vi "Get Device Channels.vi"(8 "error in":errorcluster, 11 "Device Reference in":T1 format="%.0x") -> (0 "error out":errorcluster, 2 "Device Channels":T2 {"Status"."BD Refs"."Data Reference" format="%.0x"; "Command"."BD Refs"."Data Reference" format="%.0x"}, 3 "Device Reference out":T1 format="%.0x")   [LabVIEW 2020, in "SEECD Engine.lvlib"]
uses:
  SEECD Engine.lvlib
  <vilib>/NI VeriStand/Custom Device API/Custom Device Item Ref.ctl
  Type Defs/Device Channels.ctl
  Type Defs/Output Data.ctl
  <vilib>/NI VeriStand/Custom Device API/Block Data Reference.ctl
  <vilib>/NI VeriStand/Custom Device API/Data Reference.ctl
  Type Defs/Input Data.ctl
  Type Defs/Data Ref FGV Command.ctl
  <vilib>/NI VeriStand/Custom Device API/Custom Device Channel Type.ctl
  <vilib>/NI VeriStand/Custom Device API/Data Access Type.ctl
  <vilib>/NI VeriStand/Custom Device Tools/Custom Device Utility Library/NI VeriStand - Search for Item by Name.vi
  <vilib>/NI VeriStand/Custom Device Tools/Custom Device Utility Library/Custom Device Utility Library.lvlib
  <vilib>/NI VeriStand/Custom Device API/Custom Device API.lvlib
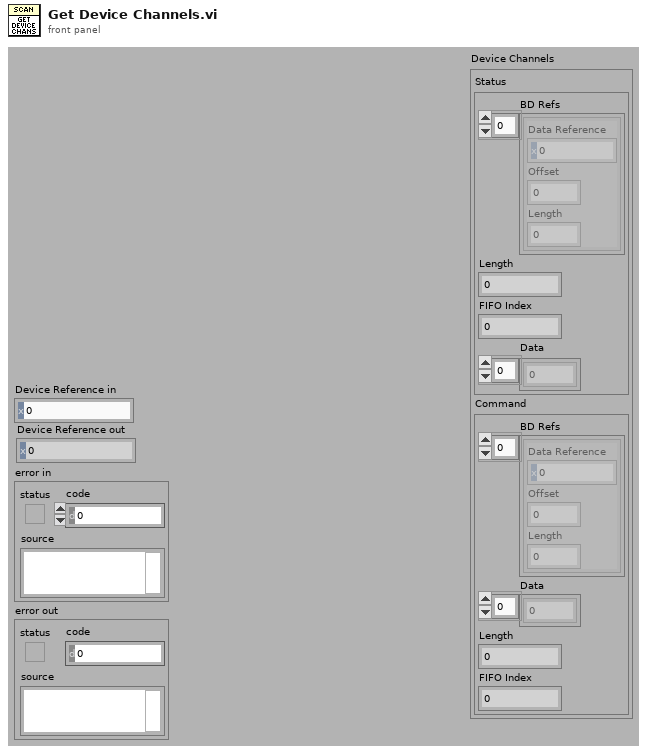
[diagram p1: front panel]
types:
  T1 = typedef "Custom Device API.lvlib/Custom Device Item Ref.ctl" = u64
  T2 = typedef "SEECD Engine.lvlib/Device Channels.ctl" = cluster{"Status":T3, "Command":T6}
  T3 = typedef "SEECD Engine.lvlib/Output Data.ctl" = cluster{"BD Refs":T4[], "Length":i32, "FIFO Index":i32, "Data":dbl[]}
  T4 = typedef "Custom Device API.lvlib/Block Data Reference.ctl" = cluster{"Data Reference":T5, "Offset":u64, "Length":u64}
  T5 = typedef "Custom Device API.lvlib/Data Reference.ctl" = i32
  T6 = typedef "SEECD Engine.lvlib/Input Data.ctl" = cluster{"BD Refs":T4[], "Data":dbl[], "Length":i32, "FIFO Index":i32}
  T7 = typedef "SEECD Engine.lvlib/Data Ref FGV Command.ctl" = enum16{"Intialize", "Get", "Update"}
  T8 = typedef "Custom Device API.lvlib/Data Access Type.ctl" = enum16{"Read", "Write"}
  T9 = typedef "Custom Device API.lvlib/Custom Device Channel Type.ctl" = enum16{"Input", "Output"}
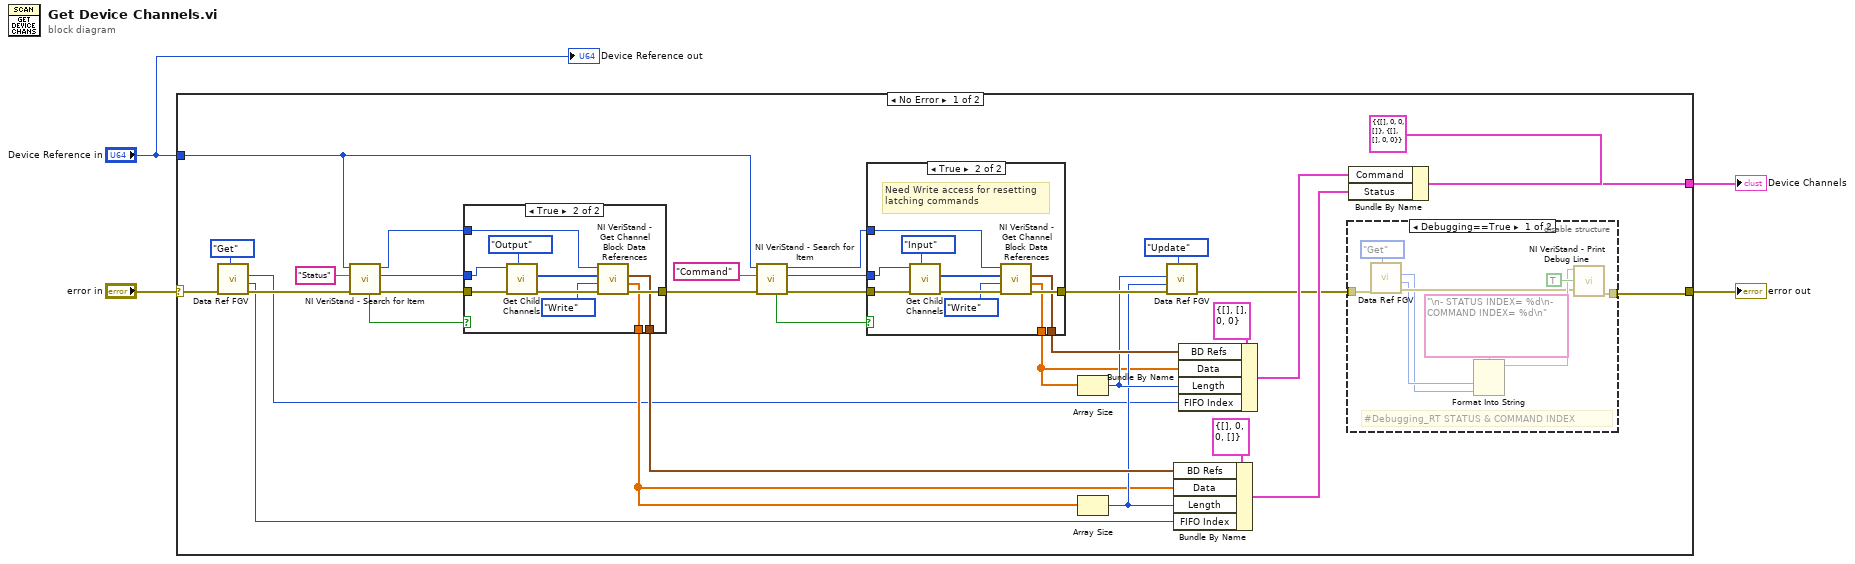
[diagram p0: block diagram]
diagram:
  n1 = case shown="No Error" "error in" {
    selector: "error in" -> [w28 w70]
    tunnel: [w5 w70] -> w3
    tunnel: "Device Reference in" -> [w31 _]
    tunnel: [w29 _] -> w1
    frame No Error {
      n2 = call "Data Ref FGV.vi"("Command"=Data_Ref_FGV_Command."Get", "error in (no error)"=w28) -> ("error out"=w27:errorcluster, "Output FIFO Index / Length"=w8:i32, "Input FIFO Index / Length"=w7:i32)  [unwired: 6 in, 1 out]
      n3 = call-poly <vilib>:"NI VeriStand - Search for Item.vi"("error in"=w27, "Item Name"="Status" ("Section Name"), "Section Ref in"=w31) -> ("error out"=w34:errorcluster, "Item Ref"=w35:T1, "Section Ref out"=w25:T1, "Found"=w36:bool)  [unwired: 5 in]
      n4 = case shown="True" w36 {
        tunnel: w35 -> [_ w68]
        tunnel: w34 -> [w59 w67]
        tunnel: [w59 w65] -> w30
        tunnel: w25 -> [_ w63]
        tunnel: [_ w61] -> w10
        tunnel: [_ w60] -> w18
        frame False {
        }
        frame True {
          n5 = call "Get Child Channels.vi"("Channel Type"=Custom_Device_Channel_Type."Output", "error in"=w67, "Section Ref in"=w68) -> ("error out"=w66:errorcluster, "Channel Refs"=w64:T1[])  [unwired: 5 in, 2 out]
          n6 = call <vilib>:"NI VeriStand - Get Channel Block Data References.vi"("error in (no error)"=w66, "Access"=Data_Access_Type."Write", "Channel Refs"=w64, "Device Ref in"=w63) -> ("error out"=w65:errorcluster, "Values Array"=w61:dbl[], "Block Data Refs"=w60:T4[])  [unwired: 4 in, 1 out]
        }
      }
      n7 = call-poly <vilib>:"NI VeriStand - Search for Item.vi"("error in"=w30, "Item Name"="Command" ("Section Name"), "Section Ref in"=w31) -> ("error out"=w23:errorcluster, "Item Ref"=w22:T1, "Section Ref out"=w21:T1, "Found"=w24:bool)  [unwired: 5 in]
      n8 = case shown="True" w24 {
        tunnel: w22 -> [_ w57]
        tunnel: w23 -> [w48 w56]
        tunnel: [w48 w54] -> w19
        tunnel: w21 -> [_ w52]
        tunnel: [_ w50] -> w9
        tunnel: [_ w49] -> w17
        frame False {
        }
        frame True {
          # "Need Write access for resetting\nlatching commands"
          n9 = call "Get Child Channels.vi"("Channel Type"=Custom_Device_Channel_Type."Input", "error in"=w56, "Section Ref in"=w57) -> ("error out"=w55:errorcluster, "Channel Refs"=w53:T1[])  [unwired: 5 in, 2 out]
          n10 = call <vilib>:"NI VeriStand - Get Channel Block Data References.vi"("error in (no error)"=w55, "Access"=Data_Access_Type."Write", "Channel Refs"=w53, "Device Ref in"=w52) -> ("error out"=w54:errorcluster, "Values Array"=w50:dbl[], "Block Data Refs"=w49:T4[])  [unwired: 4 in, 1 out]
        }
      }
      n11 = Array Size(array=w9) -> (size(s)=w12:i32)
      n12 = Array Size(array=w10) -> (size(s)=w11:i32)
      n13 = call "Data Ref FGV.vi"("Command"=Data_Ref_FGV_Command."Update", "error in (no error)"=w19, "Output Length"=w11, "Input Length"=w12) -> ("error out"=w6:errorcluster)  [unwired: 4 in, 3 out]
      n14 = Bundle By Name(cluster=T3 {"BD Refs"=[], "Length"=0, "FIFO Index"=0, "Data"=[]} ("Output Data"), "BD Refs"=w18, "Data"=w10, "Length"=w11, "FIFO Index"=w8) -> (w13:T3)
      n15 = Bundle By Name(cluster=T6 {"BD Refs"=[], "Data"=[], "Length"=0, "FIFO Index"=0} ("Input Data"), "BD Refs"=w17, "Data"=w9, "Length"=w12, "FIFO Index"=w7) -> (w14:T6)
      n16 = disable-structure shown="Debugging==True" {
        disable-tunnel: w6 -> [w46 w47]
        disable-tunnel: [w40 w47] -> w5
        frame condition #0 {
          # "#Debugging_RT STATUS & COMMAND INDEX"
          n17 = call "Data Ref FGV.vi"("Command"=Data_Ref_FGV_Command."Get", "error in (no error)"=w46) -> ("error out"=w41:errorcluster, "Output FIFO Index / Length"=w39:i32, "Input FIFO Index / Length"=w38:i32)  [unwired: 6 in, 1 out]
          n18 = Format Into String(format string="\n- STATUS INDEX= %d\n- COMMAND INDEX= %d\n", w39, w38) -> (resulting string=w42:string)  [unwired: 2 in, 1 out]
          n19 = call <vilib>:"NI VeriStand - Print Debug Line.vi"("error in (no error)"=w41, "Add to log file? (F)"=TRUE, "Message"=w42) -> ("error out"=w40:errorcluster)  [unwired: 8 in]
        }
        frame condition #1 (active) {
        }
      }
      n20 = Bundle By Name(cluster=T2 {"Status"={"BD Refs"=[], "Length"=0, "FIFO Index"=0, "Data"=[]}, "Command"={"BD Refs"=[], "Data"=[], "Length"=0, "FIFO Index"=0}} ("Device Channels"), "Command"=w14, "Status"=w13) -> (w29:T2)
    }
    frame Error {
    }
  }
  "Device Channels" <- w1
  "error out" <- w3
  "Device Reference out" <- "Device Reference in"
